vi "niFPGA Shift 1 Saturate (I64 to 16).vi"(2 "I64 input":i64 format="%08x") -> (6 "saturated I16 output":i16 format="%.0x")   [LabVIEW 2017]
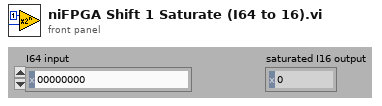
[diagram p1: front panel]
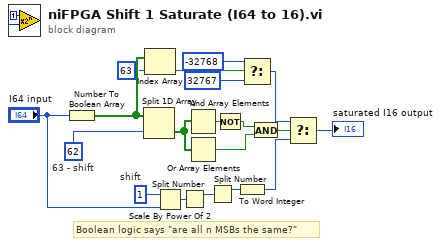
[diagram p0: block diagram]
diagram:
  w19 = i8 1  # shift
  w18 = i8 62  # 63 - shift
  # "Boolean logic says \"are all n MSBs the same?\""
  n1 = Number To Boolean Array(number="I64 input") -> (Boolean array=w14:bool[])
  n2 = Split 1D Array(array=w14, index=w18) -> (second subarray=w15:bool[])  [unwired: 1 out]
  n3 = Index Array(array=w14, index=63) -> (element=w12:bool)
  n4 = Scale By Power Of 2(n=w19, x="I64 input") -> (x*2^n=w16:i64)
  n5 = Split Number(x=w16) -> (hi(x)=w2:u32)  [unwired: 1 out]
  n6 = And Array Elements(Boolean array=w15) -> (logical AND=w8:bool)
  n7 = Or Array Elements(Boolean array=w15) -> (logical OR=w6:bool)
  n8 = Split Number(x=w2) -> (hi(x)=w1:u16)  [unwired: 1 out]
  n9 = Not(x=w8) -> (.not. x?=w7:bool)
  n10 = To Word Integer(number=w1) -> (16bit integer=w3:i16)
  n11 = Select(t=i16 -32768, s=w12, f=i16 32767) -> (s? t:f=w4:i16)
  n12 = And(x=w7, y=w6) -> (x .and. y?=w5:bool)
  n13 = Select(t=w4, s=w5, f=w3) -> (s? t:f=→"saturated I16 output":i16)
